vi "synnax channel retrieve keys.vi"(7 "handle":u64, 8 "error in (no error)":errorcluster, 10 "count":u64, 11 "name(s)":string) -> (0 "error out":errorcluster, 1 "out_index_keys":u32[](array[numeric]), 2 "out_dtypes":string[](array[numeric]), 3 "out_keys":u32[](array[numeric]))   [LabVIEW 2026, in "synnax_clib.lvlib" / "Synnax Client.lvclass"]
uses:
  Synnax Client.lvclass
  Synnax Client.lvclass/Synnax Client.ctl
  synnax_clib.lvlib
  synnax_clib.dll
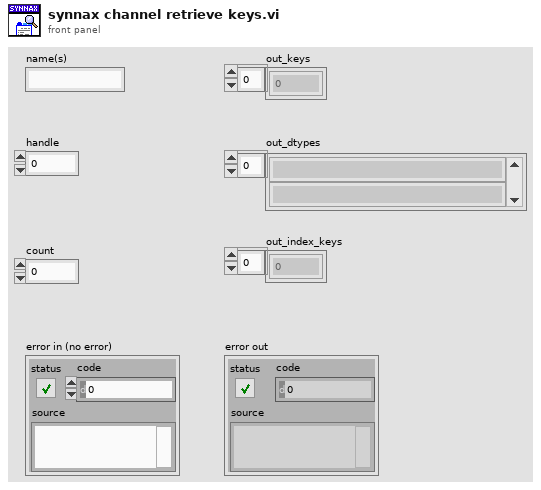
[diagram p1: front panel]
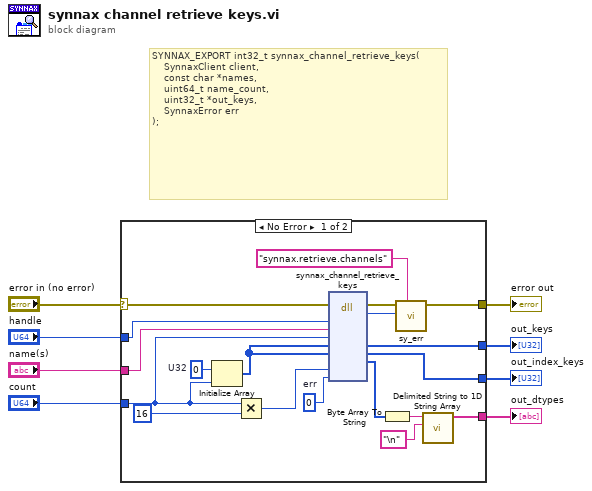
[diagram p0: block diagram]
diagram:
  # "SYNNAX_EXPORT int32_t synnax_channel_retrieve_keys(\n    SynnaxClient client,\n    const char *names,\n    uint64_t name_count,\n    uint32_t *out_keys,\n    SynnaxError err\n);"
  n1 = case shown="No Error" "error in (no error)" {
    selector: "error in (no error)" -> [w15 w28]
    tunnel: "handle" -> [w27 _]
    tunnel: "name(s)" -> [w26 _]
    tunnel: [w25 _] -> w6
    tunnel: [w21 w28] -> w5
    tunnel: "count" -> [w13 _]
    tunnel: [w17 _] -> w3
    tunnel: [w9 _] -> w1
    frame No Error {
      w14 = u32 0  # U32
      w24 = u64 0  # err
      n2 = Initialize Array(w14, w13) -> (w10:u32[])
      n3 = Multiply(x=w13, y=u64 16) -> (x*y=w19:u64)
      n4 = dll-call lib="C/synnax/client/labview/synnax_clib.*" fn="synnax_channel_retrieve_keys"(error in=w15, "client"=w27, "names"=w26, "name_count"=w13, "out_keys"=w10, "out_index_keys"=w10, "out_dtypes_size"=w19, "err"=w24) -> (error out=w22:errorcluster, "return type"=w20:i32, "out_keys"=w25:u32[], "out_index_keys"=w9:u32[], "out_dtypes"=w12:u8[])  [unwired: 8 in, 1 out]
      n5 = Byte Array To String(unsigned byte array=w12) -> (string=w11:string)
      n6 = call "sy_err.vi"("source"="synnax.retrieve.channels", "error code"=w20, "error in (no error)"=w22) -> ("error out"=w21:errorcluster)  [unwired: 8 in]
      n7 = call <vilib>:"Delimited String to 1D String Array.vi"("delimiter"="\n", "delimited string"=w11) -> ("string array"=w17:string[])  [unwired: 9 in]
    }
    frame Error {
    }
  }
  "out_keys" <- w6
  "error out" <- w5
  "out_dtypes" <- w3
  "out_index_keys" <- w1
